vi "Remove NaN-containing Pairs.vi"(8 "Error In":errorcluster, 9 "Y Array in":dbl[](array[numeric]), 11 "X Array in":dbl[](array[numeric])) -> (0 "Error Out":errorcluster, 1 "Y Array out":dbl[](array[numeric]), 2 "# X elts deleted":i32, 3 "X Array out":dbl[](array[numeric]))   [LabVIEW 2019]
panel:
  out "# Y elts deleted":i32
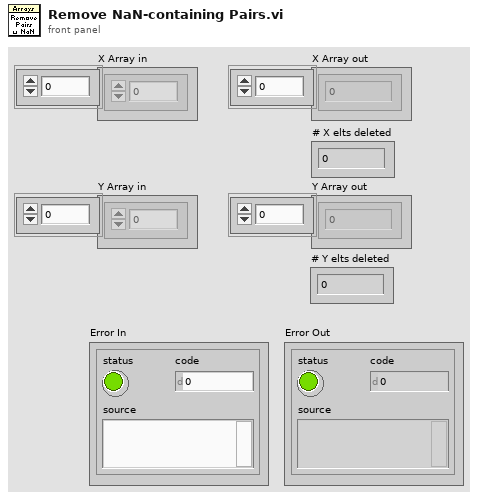
[diagram p1: front panel]
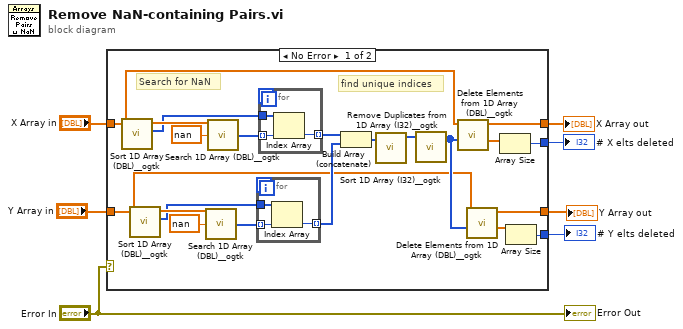
[diagram p0: block diagram]
diagram:
  n1 = case shown="No Error" "Error In" {
    tunnel: "X Array in" -> [w18 w36]
    tunnel: [w15 w36] -> w6
    tunnel: "Y Array in" -> [w13 w35]
    tunnel: [w12 w35] -> w4
    tunnel: [w10 _] -> w3
    tunnel: [w8 _] -> w2
    frame No Error {
      # "find unique indices"
      # "Search for NaN"
      n2 = call <userlib>:"Sort 1D Array (DBL)__ogtk.vi"("Array in"=w18) -> ("Sorted Pointers"=w23:i32[], "Sorted Array out"=w28:dbl[])  [unwired: 9 in]
      n3 = call <userlib>:"Sort 1D Array (DBL)__ogtk.vi"("Array in"=w13) -> ("Sorted Pointers"=w21:i32[], "Sorted Array out"=w25:dbl[])  [unwired: 9 in]
      n4 = call <userlib>:"Search 1D Array (DBL)__ogtk.vi"("Array"=w25, "Element Data"=nan ("element")) -> ("Indices of Elements"=w22:i32[])  [unwired: 7 in]
      n5 = call <userlib>:"Search 1D Array (DBL)__ogtk.vi"("Array"=w28, "Element Data"=nan ("element")) -> ("Indices of Elements"=w24:i32[])  [unwired: 7 in]
      n6 = for {
        tunnel: w22 -> [w30] mode=indexing
        tunnel: w21 -> [w31]
        tunnel: [w29] -> w19 mode=indexing
        n7 = Index Array(array=w31, index=w30) -> (element=w29:i32)
      }
      n8 = for {
        tunnel: w24 -> [w33] mode=indexing
        tunnel: w23 -> [w34]
        tunnel: [w32] -> w20 mode=indexing
        n9 = Index Array(array=w34, index=w33) -> (element=w32:i32)
      }
      n10 = Build Array (concatenate)(w20, w19) -> (w17:i32[])
      n11 = call <userlib>:"Sort 1D Array (I32)__ogtk.vi"("Array in"=w17) -> ("Sorted Array out"=w16:i32[])  [unwired: 9 in, 1 out]
      n12 = call <userlib>:"Remove Duplicates from 1D Array (I32)__ogtk.vi"("Input Array"=w16) -> ("Output Array"=w14:i32[])  [unwired: 1 out]
      n13 = call <userlib>:"Delete Elements from 1D Array (DBL)__ogtk.vi"("indices"=w14, "array"=w18) -> ("deleted elements"=w11:dbl[], "array w/ subset deleted"=w15:dbl[])  [unwired: 8 in]
      n14 = call <userlib>:"Delete Elements from 1D Array (DBL)__ogtk.vi"("indices"=w14, "array"=w13) -> ("deleted elements"=w9:dbl[], "array w/ subset deleted"=w12:dbl[])  [unwired: 8 in]
      n15 = Array Size(array=w11) -> (size(s)=w10:i32)
      n16 = Array Size(array=w9) -> (size(s)=w8:i32)
    }
    frame Error {
    }
  }
  "Y Array out" <- w4
  "X Array out" <- w6
  "# X elts deleted" <- w3
  "# Y elts deleted" <- w2
  "Error Out" <- "Error In"
